vi "Get bracketed array elements.vi"(8 "error in (no error)":errorcluster, 9 "requriedObject":string, 10 "brackettedElements":string, 11 "Variant in":variant) -> (0 "error out":errorcluster, 2 "error?":bool, 3 "Array Element":variant)   [LabVIEW 2015]
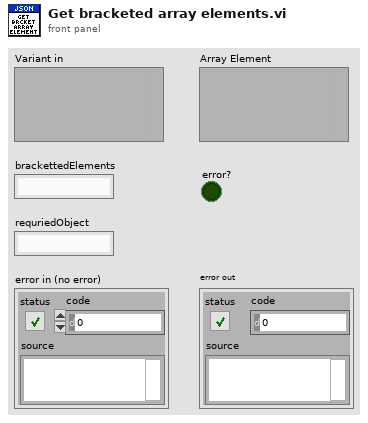
[diagram p1: front panel]
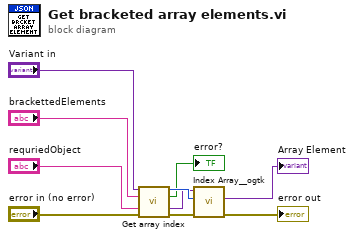
[diagram p0: block diagram]
diagram:
  n1 = call "Get array index.vi"("Variant in"="Variant in", "brackettedElements"="brackettedElements", "requriedObject"="requriedObject", "error in (no error)"="error in (no error)") -> ("indexOut"=w6:i32, "Element found?"=→"error?":bool, "VArray"=w5:variant, "error out"=w4:errorcluster)  [unwired: 5 in, 3 out]
  n2 = call <userlib>:"Index Array__ogtk.vi"("error in (no error)"=w4, "Index (1D)"=w6, "MultiD Array"=w5) -> ("error out"=→"error out":errorcluster, "Array Element"=→"Array Element":variant)  [unwired: 7 in]
